vi "Tosca-Schedule Params to Table.vi"(0 "Param Table":refnum<vi>, 2 "Name":string, 7 "Table":T1[](array[typedef])) -> ()   [LabVIEW 2020]
uses:
  epl-vi-lib/Utility VIs/Controls/KTable/KTable.xctl
  Typedefs/Tosca-Parameter Table Element.ctl
  Typedefs/Tosca-Parameter Dimension.ctl
panel:
  out "variant":variant
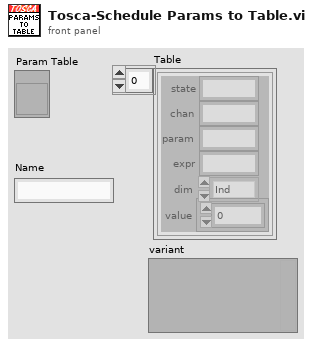
[diagram p1: front panel]
types:
  T1 = typedef "Tosca-Parameter Table Element.ctl" = cluster{"state":string, "chan":string, "param":string, "expr":string, "dim":T2, "value":dbl[]}
  T2 = typedef "Tosca-Parameter Dimension.ctl" = enum16{"Ind", "X", "Y"}
  T3 = cluster{"state":string, "chan":string, "param":string, "dim":T2, "expr":string}
  T4 = enum8{"Enabled", "Disabled", "Disabled and Grayed Out"}
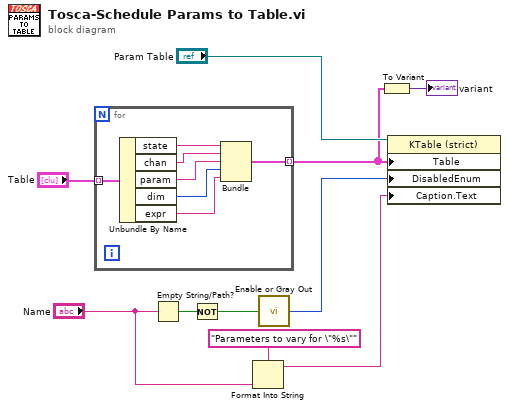
[diagram p0: block diagram]
diagram:
  n1 = for {
    tunnel: "Table" -> [w17] mode=indexing
    tunnel: [w13] -> w2 mode=indexing
    n2 = Unbundle By Name(w17) -> ("state"=w16:string, "chan"=w15:string, "param"=w14:string, "dim"=w12:T2, "expr"=w11:string)
    n3 = Bundle("state"=w16, "chan"=w15, "param"=w14, "dim"=w12, "expr"=w11) -> (w13:T3)  [unwired: 1 in]
  }
  n4 = Empty String/Path?(string/path="Name") -> (empty?=w6:bool)
  n5 = Not(x=w6) -> (.not. x?=w5:bool)
  n6 = Format Into String(format string="Parameters to vary for \"%s\"", "Name") -> (resulting string=w3:string)  [unwired: 2 in, 1 out]
  n7 = call "Enable or Gray Out.vi"("Boolean"=w5) -> ("Disabled"=w4:T4)
  n8 = To Variant(anything=w2) -> (Variant=→"variant":variant)
  n9 = property class="KTable (strict)"(reference="Param Table", "Table"=w2, "DisabledEnum"=w4, "Caption.Text"=w3) -> ()  [unwired: 1 in, 2 out]
